vi "ReadButtonPressTillStop.vi"(5 "error in (no error)":errorcluster) -> (6 "Boolean Data Read 2":bool[](array[boolean]) caption="Boolean Data Read, During", 8 "error out":errorcluster)   [LabVIEW 2015]
doc: "I. Description:\nThis example demonstrates how to read values from one or more digital input channels.\n\nII. Instructions for Running:\n1. Select the digital lines on the DAQ device to be read.\nNote: The array indicator is sized for 8 lines, if using fewer lines, not all elements will be used. Also, if using more lines, use the array index to view elements beyond the first eight lines.\n\nIII. Block Diagram Steps:\n1. Create a Digital Input channel. Use one channel for all lines. You can alternatively use one channel for each line, but then use a different polymorphic version of the DAQmx Read VI.\n2. Call the Start VI to start the task.\n3. Read the digital data in a loop until the user hits the stop button or an error occurs. This read VI reads a single sample of digital data on demand, so no timeout is necessary.\n4. Use the Boolean Array to Number VI to view the values read as a single number\n5. Call the Clear Task VI to clear the Task.\n6. Use the popup dialog box to display an error or warning if any.\n\nIV. I/O Connections Overview:\nMake sure your signal input terminals match the Lines I/O Control. In this case wire your digital signals to the first eight digital lines on your DAQ Device."
uses:
  <vilib>/DAQmx/read.llb/DAQmx Read (Digital 1D Bool 1Chan 1Samp).vi
  <vilib>/DAQmx/create/channels.llb/DAQmx Create Channel (DI-Digital Input).vi
  DAQ Engine VIs/PXI Globals.vi
  <vilib>/DAQmx/miscellaneous.llb/DAQmx Fill In Error Info.vi
panel:
  out "Hexadecimal Data Read":u32 format="%x"
  in  "Lines":tag="PXI1Slot4/port0/line4:0"
  in  "stop":bool
  # "For instructions, select Help>>Show Context Help"
  # "Channel Parameters"
  # "Bits"
  # "0"
  # "1"
  # "2"
  # "3"
  # "4"
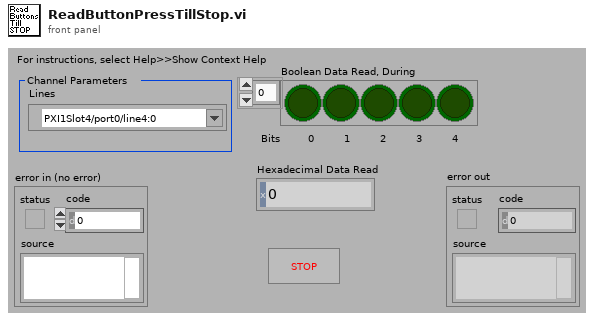
[diagram p1: front panel]
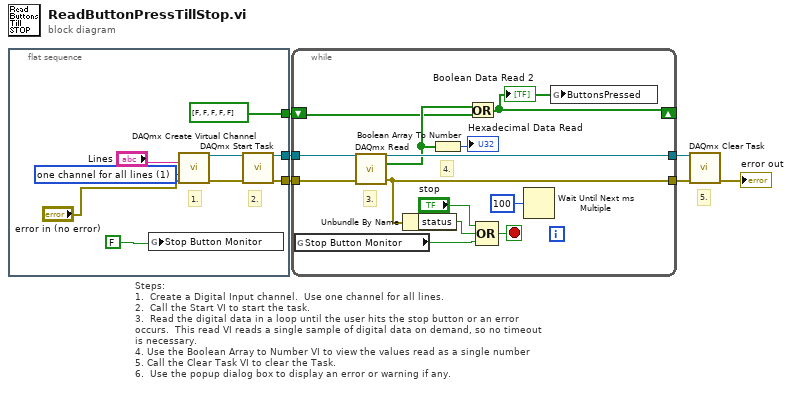
[diagram p0: block diagram]
diagram:
  # "Steps: \n1.  Create a Digital Input channel.  Use one channel for all lines.  \n2.  Call the Start VI to start the task.\n3.  Read the digital data in a loop until the user hits the stop button or an error occurs.  This read VI reads a single sample of digital data on demand, so no timeout is necessary.\n4. Use the Boolean Array to Number VI to view the values read as a single number\n5. Call the Clear Task VI to clear the Task.\n6.  Use the popup dialog box to display an error or warning if any."
  # "5."
  n1 = flat-sequence {
    tunnel: [w15] -> w6
    tunnel: [w14] -> w4
    tunnel: [bool[] [FALSE, FALSE, FALSE, FALSE, FALSE] ("Boolean Data Read 2")] -> w2
    frame #0 {
      w10 = 1 items=["one channel for each line", "one channel for all lines"] ("line grouping")
      # "2."
      # "1."
      n2 = global write "PXI Globals.vi" "Stop Button Monitor"(FALSE) -> ()
      n3 = call-poly <vilib>:"DAQmx Create Virtual Channel.vi"("lines"="Lines", "line grouping"=w10, "error in"="error in (no error)") -> ("task out"=w13:refnum<k21>, "error out"=w12:errorcluster)  [unwired: 11 in]
      n4 = call <vilib>:"DAQmx Start Task.vi"("task/channels in"=w13, "error in"=w12) -> ("task out"=w14:refnum<k21>, "error out"=w15:errorcluster)  [unwired: 12 in]
    }
  }
  n5 = while {
    tunnel: w6 -> [w28]
    tunnel: [w25] -> w5
    tunnel: w4 -> [w24]
    tunnel: [w23] -> w3
    shift-right: [w16] -> _
    shift-left: w2 -> [w19]
    stop <- w27 stop-if-true
    # "4."
    # "3."
    n6 = global read "PXI Globals.vi" "Stop Button Monitor"() -> (w18:bool)
    n7 = call-poly <vilib>:"DAQmx Read.vi"("task/channels in"=w24, "error in"=w28) -> ("task out"=w23:refnum<k21>, "data"=w20:bool[], "error out"=w25:errorcluster)  [unwired: 11 in]
    n8 = Unbundle By Name(w25) -> ("status"=w26:bool)
    n9 = Boolean Array To Number(Boolean array=w20) -> (number=→"Hexadecimal Data Read":u32)
    n10 = Or(x=w20, y=w19) -> (x .or. y?=w16:bool[])
    "Boolean Data Read 2" <- w16
    n11 = Compound Arithmetic op=OR("stop", w26, w18) -> (w27:bool)
    n12 = Wait Until Next ms Multiple(millisecond multiple=u32 100 ("milliseconds to wait")) -> ()  [unwired: 1 out]
    n13 = global write "PXI Globals.vi" "ButtonsPressed"(w16) -> ()
  }
  n14 = call <vilib>:"DAQmx Clear Task.vi"("task in"=w3, "error in"=w5) -> ("error out"=→"error out":errorcluster)  [unwired: 13 in]
